vi "VisionSimulationExecute.v.vi"(8 "error in (no error)":errorcluster) -> (0 "error out":errorcluster)   [LabVIEW 2023]
uses:
  <vilib>/Rock Robotics/WPI/ThirdParty/JAS_Junk/TrajLib/VI/Util_GetTime_U32.vi
  <vilib>/Rock Robotics/WPI/ThirdParty/JAS_Junk/TrajLib/VI/TimeInterpDouble_New.vi
  <vilib>/Rock Robotics/WPI/ThirdParty/JAS_Junk/TrajLib/VI/TimeInterpDouble_AddSample.vi
  <vilib>/Rock Robotics/WPI/ThirdParty/JAS_Junk/TrajLib/VI/TimeInterpDouble_GetSample.vi
  <vilib>/Rock Robotics/WPI/ThirdParty/JAS_Junk/TrajLib/VI/TimeInterpDouble_SetMaxTime.vi
  <vilib>/Rock Robotics/WPI/ThirdParty/JAS_Junk/TrajLib/Timer_New.vi
  <vilib>/Rock Robotics/WPI/ThirdParty/JAS_Junk/TrajLib/VI/TimeInterpDouble_CleanUp.vi
  <vilib>/Rock Robotics/WPI/ThirdParty/JAS_Junk/TrajLib/MathUtil_Interpolate.vi
  <vilib>/Rock Robotics/WPI/ThirdParty/JAS_Junk/TrajLib/MathUtil_Clamp.vi
  <vilib>/Rock Robotics/WPI/ThirdParty/JAS_Junk/TrajLib/VI/Util_GetTime_U64.vi
  Vision/VisionGlobal.vi
  Robot Global Data.vi
  SimulateDrive/SIM_Drive_Globals.vi
  <vilib>/Utility/semaphor.llb/Obtain Semaphore Reference.vi
  <vilib>/Rock Robotics/WPI/ThirdParty/JAS_Junk/TrajLib/Timer_Reset.vi
  <vilib>/Rock Robotics/WPI/ThirdParty/JAS_Junk/TrajLib/Timer_Start.vi
  <vilib>/Rock Robotics/WPI/ThirdParty/JAS_Junk/TrajLib/Timer_Stop.vi
  <vilib>/Rock Robotics/WPI/ThirdParty/JAS_Junk/TrajLib/Timer_HasPeriodPassedOnce.vi
  <vilib>/gmath/interp.llb/Search Ordered Table.vi
  <vilib>/Rock Robotics/WPI/ThirdParty/JAS_Junk/TrajLib/Trajectory_Library.lvlib
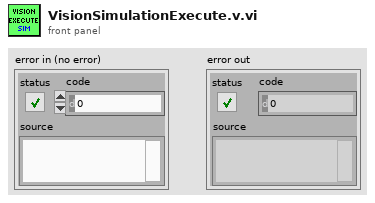
[diagram p1: front panel]
types:
  T1 = typedef "Trajectory_Library.lvlib/POSE2D.ctl" = cluster{"TRANSLATION":T2, "ROTATION":T3}
  T2 = typedef "Trajectory_Library.lvlib/TRANSLATION2D.ctl" = cluster{"X":dbl, "Y":dbl}
  T3 = typedef "Trajectory_Library.lvlib/ROTATION2D.ctl" = cluster{"VALUE":dbl, "COS":dbl, "SIN":dbl}
  T4 = typedef "Trajectory_Library.lvlib/SWERVE_DRIVE_KINEMATICS.ctl" = cluster{"NumModules":i32, "InverseKinematics":T5, "ForwardKinematics":T5, "Modules":T2[], "PrevCoR":T2, "SavedModuleStates":T6[]}
  T5 = typedef "NI_Matrix.lvlib/RealMatrix.ctl" = dbl[][]
  T6 = typedef "Trajectory_Library.lvlib/SWERVE_DRIVE_MODULE_STATE.ctl" = cluster{"Speed":dbl, "Angle":T3}
  T7 = typedef "Trajectory_Library.lvlib/SWERVE_DRIVE_MODULE_POSITION.ctl" = cluster{"Distance":dbl, "Angle":T3, "P":bool}
  T8 = typedef "Trajectory_Library.lvlib/SWERVE_DRIVE_POSE_EST2_CONFIG.ctl" = cluster{"Wheel_Locations M":T2[], "Odom X std dev M":dbl, "Odom Y std dev M":dbl, "Odom Heading std dev Rad":dbl, "Vision X std dev M":dbl, "Vision Y std dev M":dbl, "Vision Heading std dev Rad":dbl}
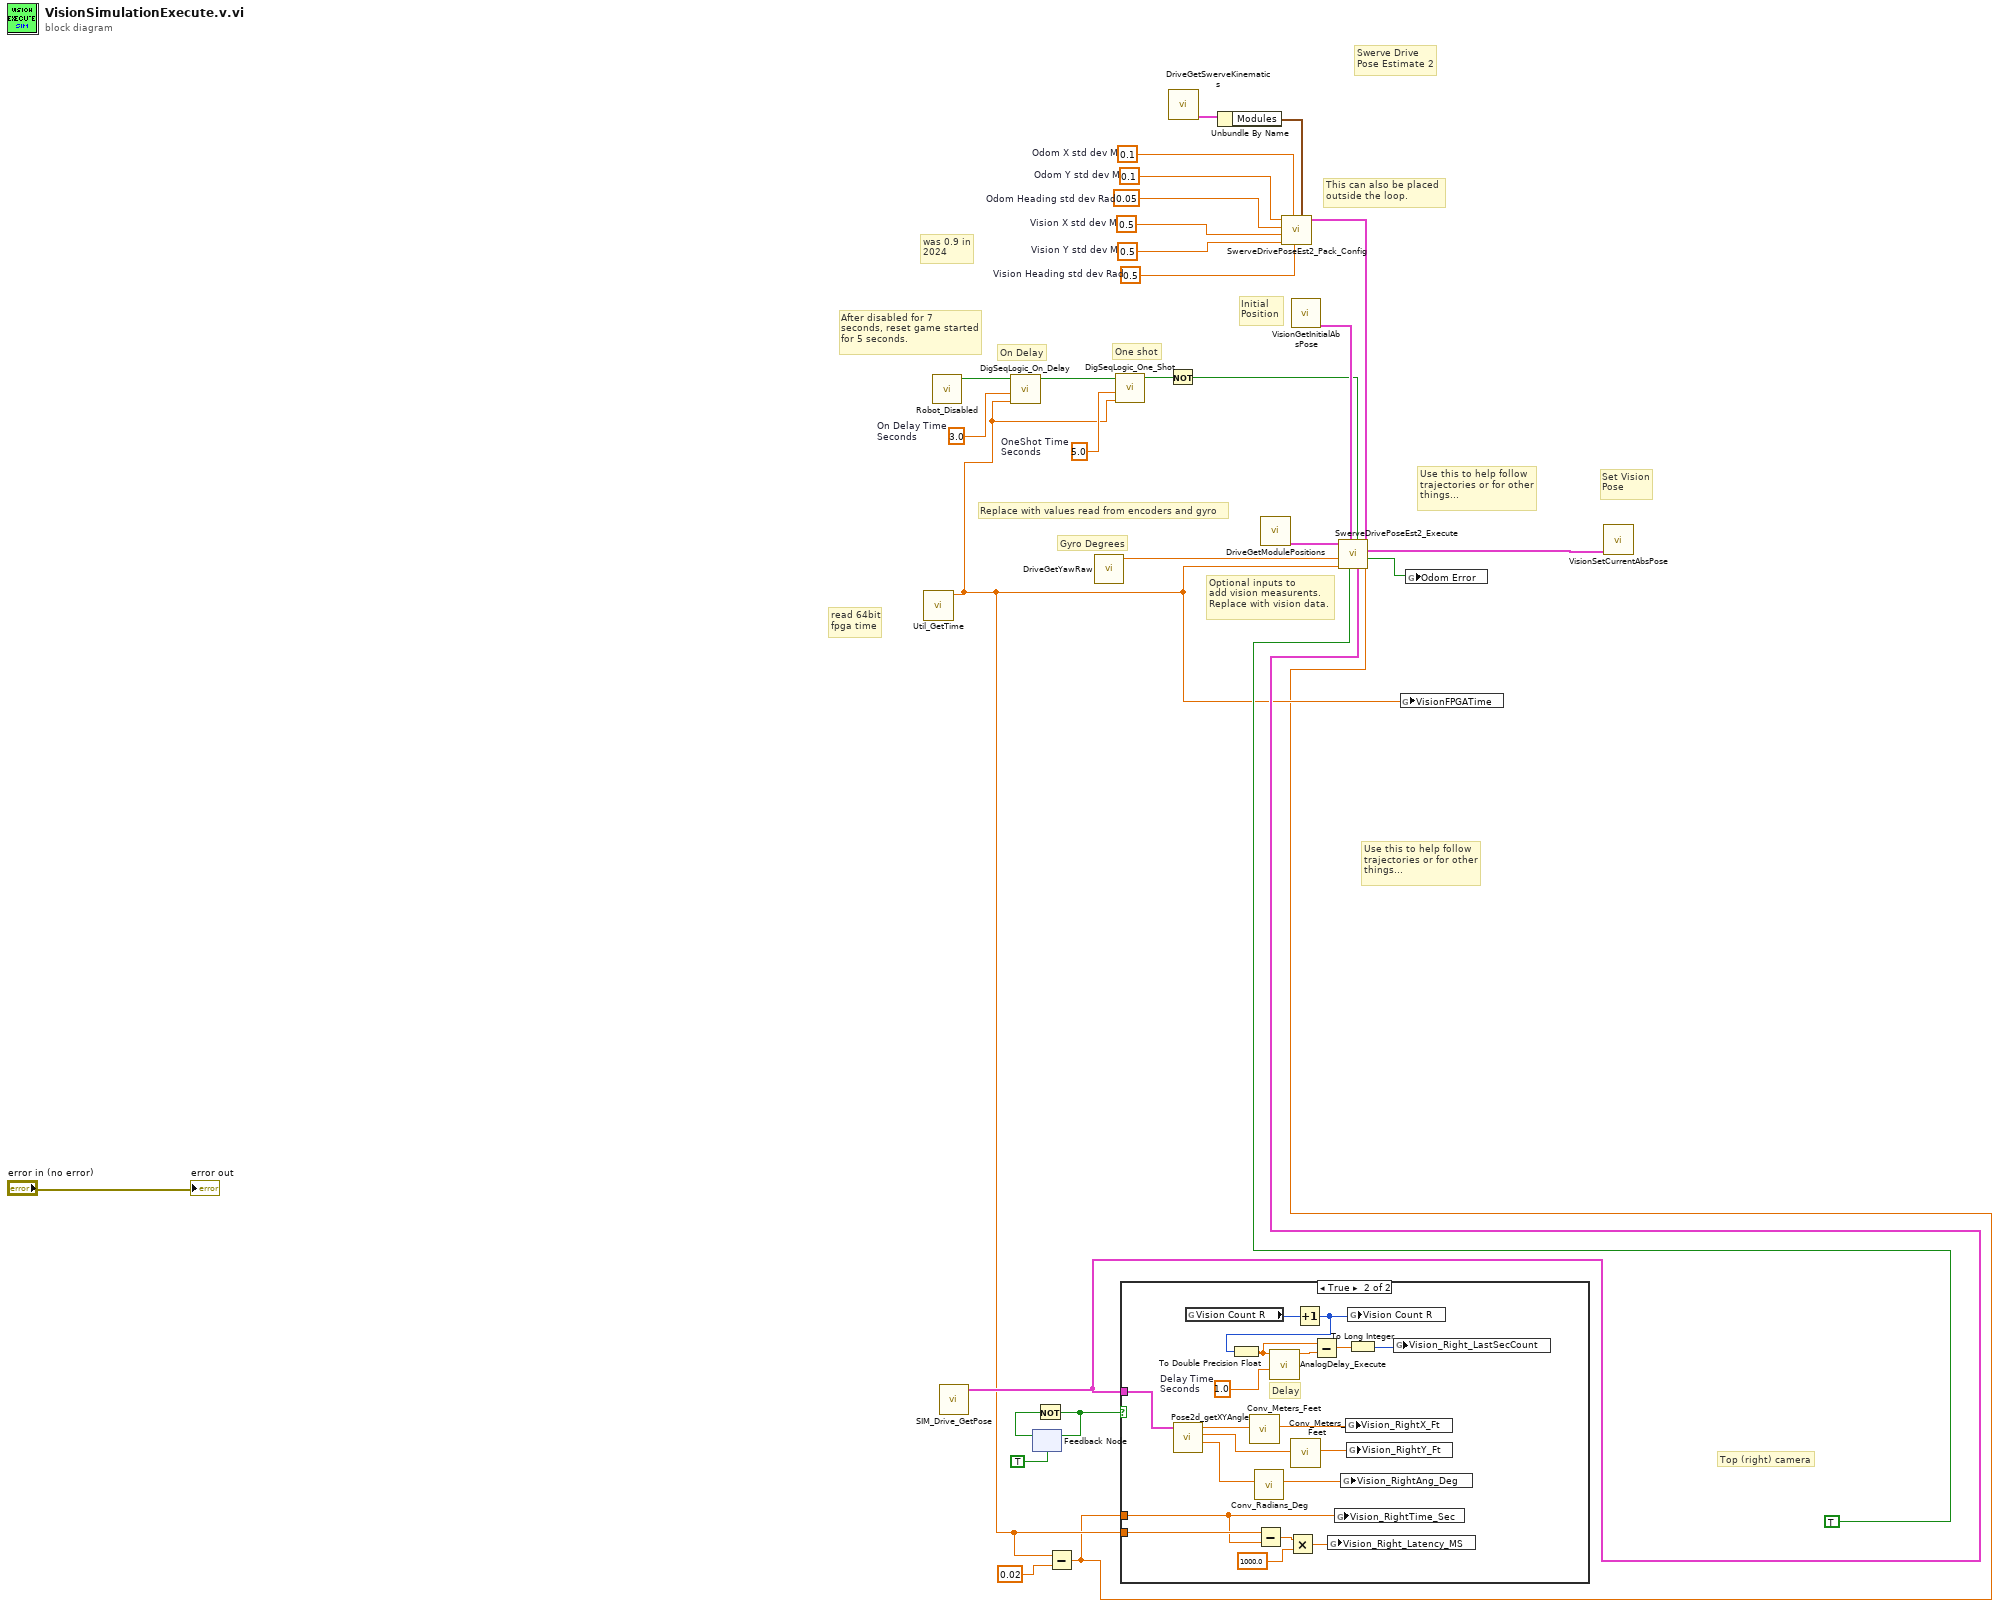
[diagram p0: block diagram]
diagram:
  w11 = 5.0  # OneShot Time Seconds
  w13 = 3.0  # On Delay Time Seconds
  w24 = 0.1  # Odom Y std dev M
  w25 = 0.05  # Odom Heading std dev Rad
  w26 = 0.5  # Vision X std dev M
  w27 = 0.5  # Vision Y std dev M
  w28 = 0.1  # Odom X std dev M
  w29 = 0.5  # Vision Heading std dev Rad
  # "Top (right) camera"
  # "Set Vision\nPose"
  # "After disabled for 7\nseconds, reset game started\nfor 5 seconds."
  # "One shot"
  # "On Delay"
  # "was 0.9 in\n2024"
  # "Initial\nPosition"
  # "Optional inputs to\nadd vision measurents.\nReplace with vision data."
  # "Replace with values read from encoders and gyro"
  # "read 64bit\nfpga time"
  # "This can also be placed \noutside the loop."
  # "Use this to help follow\ntrajectories or for other\nthings..."
  # "Swerve Drive \nPose Estimate 2"
  # "Use this to help follow\ntrajectories or for other\nthings..."
  # "Gyro Degrees"
  n1 = call <vilib>:"Util_GetTime.vi"() -> ("FPGA_Time_Seconds"=w6:dbl)  [unwired: 9 in, 2 out]
  n2 = call "Robot_Disabled.vi"() -> ("Robot Disabled"=w12:bool)  [unwired: 11 in]
  n3 = call "SIM_Drive_GetPose.vi"() -> ("POSE"=w18:T1)  [unwired: 11 in]
  n4 = call <vilib>:"DigSeqLogic_On_Delay.vi"("Time"=w6, "Delay"=w13, "Input"=w12) -> ("Output"=w10:bool)  [unwired: 7 in, 1 out]
  n5 = feedback #1(TRUE) -> (w1:bool)
  n6 = Not(x=w1) -> (.not. x?=w2:bool)
  n7 = feedback-in #1(w2) -> ()
  n8 = Subtract(x=w6, y=0.02) -> (x-y=w4:dbl)
  n9 = call "DriveGetYawRaw.vi"() -> ("YawRaw"=w19:dbl)  [unwired: 11 in]
  n10 = call <vilib>:"DigSeqLogic_One_Shot.vi"("Time"=w6, "OneShot"=w11, "Input"=w10) -> ("Output"=w9:bool)  [unwired: 7 in, 1 out]
  n11 = case shown="True" w2 {
    tunnel: w18 -> [_ w47]
    tunnel: w4 -> [_ w39]
    tunnel: w6 -> [_ w40]
    frame False {
    }
    frame True {
      w35 = 1.0  # Delay Time Seconds
      # "Delay"
      n12 = call <vilib>:"Pose2d_getXYAngle.vi"("in POSE"=w47) -> ("Angle"=w44:dbl, "Y"=w45:dbl, "X"=w46:dbl)  [unwired: 8 in]
      n13 = global read "VisionGlobal.vi" "Vision Count R"() -> (w48:i32)
      n14 = call <vilib>:"Conv_Meters_Feet.vi"("Meters"=w46) -> ("Feet"=w43:dbl)  [unwired: 10 in]
      n15 = call <vilib>:"Conv_Radians_Deg.vi"("Radians"=w44) -> ("Degrees"=w41:dbl)  [unwired: 10 in]
      n16 = Subtract(x=w40, y=w39) -> (x-y=w38:dbl)
      n17 = Multiply(x=w38, y=1000.0) -> (x*y=w36:dbl)
      n18 = call <vilib>:"Conv_Meters_Feet.vi"("Meters"=w45) -> ("Feet"=w42:dbl)  [unwired: 10 in]
      n19 = Increment(x=w48) -> (x+1=w31:i32)
      n20 = To Double Precision Float(number=w31) -> (double precision float=w33:dbl)
      n21 = call <vilib>:"AnalogDelay_Execute.vi"("Delay Time"=w35, "Input"=w33) -> ("Output"=w34:dbl)  [unwired: 8 in, 1 out]
      n22 = Subtract(x=w33, y=w34) -> (x-y=w32:dbl)
      n23 = global write "VisionGlobal.vi" "Vision_Right_Latency_MS"(w36) -> ()
      n24 = global write "VisionGlobal.vi" "Vision_RightTime_Sec"(w39) -> ()
      n25 = global write "VisionGlobal.vi" "Vision_RightAng_Deg"(w41) -> ()
      n26 = global write "VisionGlobal.vi" "Vision_RightX_Ft"(w43) -> ()
      n27 = global write "VisionGlobal.vi" "Vision_RightY_Ft"(w42) -> ()
      n28 = global write "VisionGlobal.vi" "Vision Count R"(w31) -> ()
      n29 = To Long Integer(number=w32) -> (32bit integer=w30:i32)
      n30 = global write "VisionGlobal.vi" "Vision_Right_LastSecCount"(w30) -> ()
    }
  }
  n31 = Not(x=w9) -> (.not. x?=w8:bool)
  n32 = call "DriveGetSwerveKinematics.vi"() -> ("SWERVE_DRIVE_KINEMATICS"=w17:T4)  [unwired: 11 in]
  n33 = Unbundle By Name(w17) -> ("Modules"=w16:T2[])
  n34 = call "DriveGetModulePositions.vi"() -> ("Swerve_Drive_Modual_Positions"=w20:T7[])  [unwired: 11 in]
  n35 = call <vilib>:"SwerveDrivePoseEst2_Pack_Config.vi"("Wheel_Locations M"=w16, "Vision Heading std dev Rad"=w29, "Odom X std dev M"=w28, "Vision Y std dev M"=w27, "Vision X std dev M"=w26, "Odom Heading std dev Rad"=w25, "Odom Y std dev M"=w24) -> ("SwervePoseEst2Config"=w23:T8)  [unwired: 4 in]
  n36 = call "VisionGetInitialAbsPose.vi"() -> ("InitialABSPose"=w14:T1)  [unwired: 10 in]
  n37 = call <vilib>:"SwerveDrivePoseEst2_Execute.vi"("Vision TImeStamp_Seconds"=w4, "SwervePoseEst2Config"=w23, "visionRobotPose"=w18, "Game Started"=w8, "Add Vision Meas"=TRUE ("Found"), "InitialPose"=w14, "Pass Through Time"=w6, "Gyro Degrees"=w19, "Module Positions"=w20) -> ("Error"=w21:bool, "Estimated Pose"=w22:T1)  [unwired: 1 in]
  n38 = global write "VisionGlobal.vi" "VisionFPGATime"(w6) -> ()
  n39 = global write "VisionGlobal.vi" "Odom Error"(w21) -> ()
  n40 = call "VisionSetCurrentAbsPose.vi"("Current ABS Pose"=w22) -> ()  [unwired: 11 in]
  "error out" <- "error in (no error)"
